vi "Register gRPC Methods.vi"(8 "error in (no error)":errorcluster, 11 "Template Server in":refnum<class "iService.lvclass">) -> (0 "error out":errorcluster, 3 "Template Server out":refnum<class "iService.lvclass">)   [LabVIEW 2019, in "gRPC-servicer.lvlib" / "iService.lvclass"]
uses:
  iService.lvclass
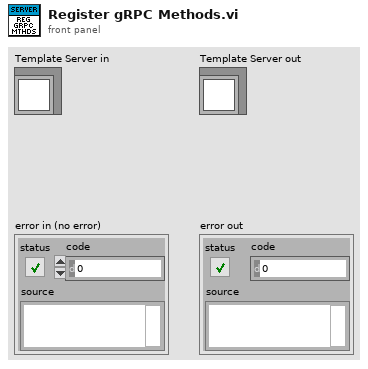
[diagram p1: front panel]
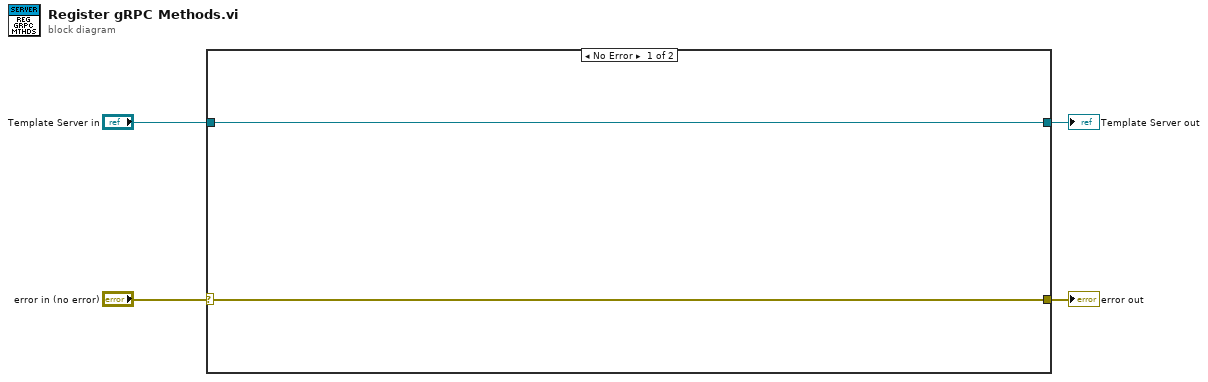
[diagram p0: block diagram]
diagram:
  n1 = case shown="No Error" "error in (no error)" {
    selector: "error in (no error)" -> [w5 w7]
    tunnel: "Template Server in" -> [w6 w8]
    tunnel: [w5 w7] -> w3
    tunnel: [w6 w8] -> w2
    frame No Error {
    }
    frame Error {
    }
  }
  "error out" <- w3
  "Template Server out" <- w2
